vi "Autonomous Mode Bool.vi"   [LabVIEW 2016]
uses:
  Globale Variable/Globale Variable.vi
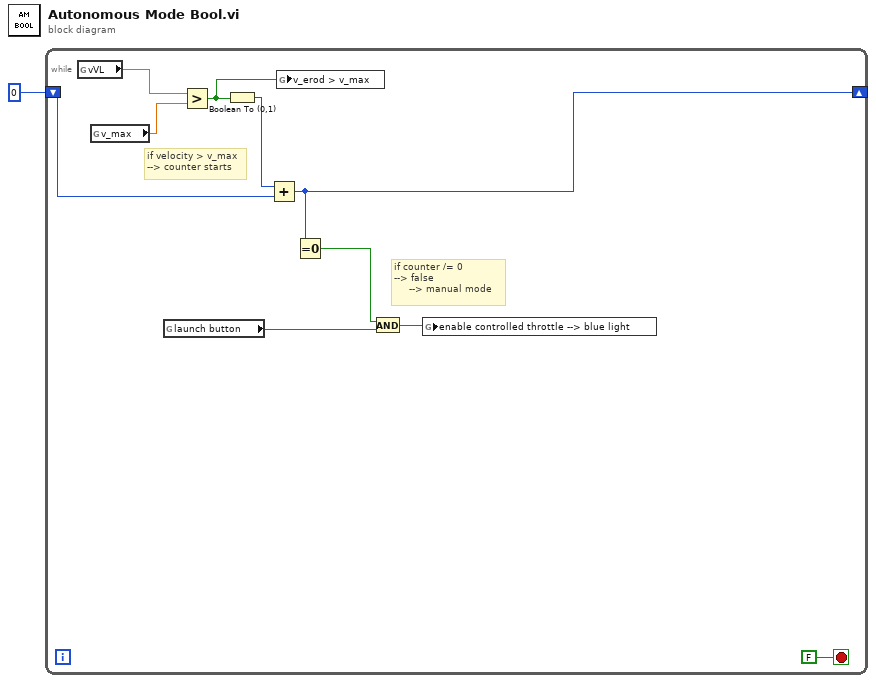
[diagram p0: block diagram]
diagram:
  n1 = while {
    shift-right: [w5] -> _
    shift-left: i16 0 -> [w9]
    stop <- FALSE stop-if-true
    # "if counter /= 0\n--> false \n     --> manual mode"
    # "if velocity > v_max\n--> counter starts"
    n2 = global read "Globale Variable.vi" "vVL"() -> (w2:dbl)
    n3 = global read "Globale Variable.vi" "v_max"() -> (w11:dbl)
    n4 = global read "Globale Variable.vi" "launch button"() -> (w4:bool)
    n5 = Greater?(x=w2, y=w11) -> (0:w3:bool)
    n6 = Boolean To (0,1)(Boolean=w3) -> (0, 1=w10:i16)
    n7 = Add(x=w10, y=w9) -> (x+y=w5:i16)
    n8 = global write "Globale Variable.vi" "v_erod > v_max"(w3) -> ()
    n9 = Equal To 0?(x=w5) -> (x = 0?=w8:bool)
    n10 = And(x=w8, y=w4) -> (x .and. y?=w7:bool)
    n11 = global write "Globale Variable.vi" "enable controlled throttle --> blue light"(w7) -> ()
  }
